vi "Get Client Operation.vi"(8 "error in (no error)":errorcluster, 11 "Identify in":refnum<class "Identify.lvclass">) -> (0 "error out":errorcluster, 2 "Client Operation":T1, 3 "Identify out":refnum<class "Identify.lvclass">)   [LabVIEW 2022 SP3, in "obs-websocket-lv.lvlib" / "Identify.lvclass"]
uses:
  Identify.lvclass
  Identify.lvclass/Identify.ctl
  Client Operation.ctl
  obs-websocket-lv.lvlib
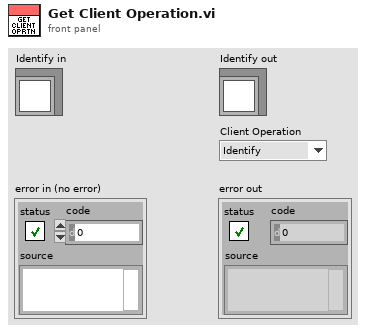
[diagram p1: front panel]
types:
  T1 = typedef "obs-websocket-lv.lvlib/Client Operation.ctl" = enum16{"Identify", "Reidentify", "Request", "RequestBatch"}
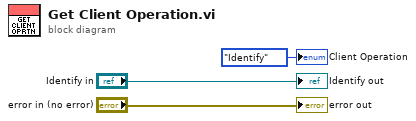
[diagram p0: block diagram]
diagram:
  "error out" <- "error in (no error)"
  "Identify out" <- "Identify in"
  "Client Operation" <- Client_Operation."Identify" ("Client Operation")
